vi "Dhoot Front Coordinate Sys.vi"(0 "Image Out":T8, 1 "First Reference ROI":T7={"Left"=660.0, "Top"=360.0, "Right"=900.0, "Bottom"=560.0, "Angle"=0.0}, 2 "Second Reference ROI":T7={"Left"=700.0, "Top"=200.0, "Right"=670.0, "Bottom"=0.0, "Angle"=0.0}, 3 "Options":T6={"Search Direction"=2, "Edge Options"={"Edge Polarity"=0, "Kernel Size"=7, "Width"=7, "Minimum Edge Strength"=40.0, "Interpolation Type"=enum."Zero Order", "Data Processing Method"=enum."Average"}, "Show Search Area"=FALSE, "Show Search Lines"=FALSE, "Show Edges Found"=FALSE, "Show Result"=TRUE, "Search Area Color"=65280, "Search Lines Color"=255, "Edge Locations Color"=16776960, "Result Color"=16711680, "Overlay Group Name"=""} {"Search Direction" items=["Left to Right", "Right to Left", "Top to Bottom", "Bottom to Top"]; "Edge Options"."Edge Polarity" items=["All Edges", "Rising Edges", "Falling Edges"]; "Edge Options"."Minimum Edge Strength" format="%.2f"; "Edge Options"."Width" step=2; "Edge Options"."Kernel Size" step=2}, 4 "Line Fit Options":T4={"Number of Lines"=1, "Type"=enum."First Edge Rake", "Min. Score"=10.0, "Max. Score"=1000.0, "Orientation"=0.0, "Angle Range"=45.0, "Angle Tolerance"=1.0, "Step Size"=7, "Min. SNR (db)"=0.0, "Min. Points (%)"=25.0, "Hough Iterations"=5} {"Min. Points (%)" min=0.0 max=100.0; "Min. SNR (db)" min=0.0; "Max. Score" min=0.0 max=1024.0; "Min. Score" min=0.0 max=1024.0 step=1.0}, 5 "error in (no error)":errorcluster, 6 "Edge Options":T1={"Edge Polarity"=0, "Kernel Size"=5, "Width"=5, "Minimum Edge Strength"=40.0, "Interpolation Type"=enum."Zero Order", "Data Processing Method"=enum."Average"} {"Edge Polarity" items=["All Edges", "Rising Edges", "Falling Edges"]; "Minimum Edge Strength" format="%.2f"; "Width" step=2; "Kernel Size" step=2}, 7 "ROI Enable True/False":bool, 8 "Step Size":u32=1, 9 "Process":T3(ring)=enum."Get First + Last Edge", 11 "Scan Direction":u16(ring) items=["Left To Right", "Right To Left", "Top To Bottom", "Bottom To Top"]) -> (13 "Angle (Pixel)":dbl, 14 "Image Out":T8, 15 "First Reference Centre":cluster{"Centre X":dbl, "Centre Y":dbl}, 16 "Second Reference Centre":cluster{"Centre X":dbl, "Centre Y":dbl}, 19 "error IO":errorcluster)   [LabVIEW 2019, in "Algorithm.lvclass"]
uses:
  FrameworkOverrides/Algorithm.lvclass
  <vilib>/vision/NI_Vision_Development_Module.lvlib
  <vilib>/vision/Image Controls.llb/IMAQ Image.ctl
  <vilib>/vision/Measure.llb/Edge Polarity.ctl
  <vilib>/vision/Measure.llb/Edge Options.ctl
  <vilib>/vision/Measure.llb/Straight Edge Process.ctl
  <vilib>/vision/Measure.llb/Straight Edge Options.ctl
panel:
  out "First ref Centre Y":dbl
  out "First ref Centre X":dbl
  out "Second ref Centre Y":dbl
  out "Second ref Centre X":dbl
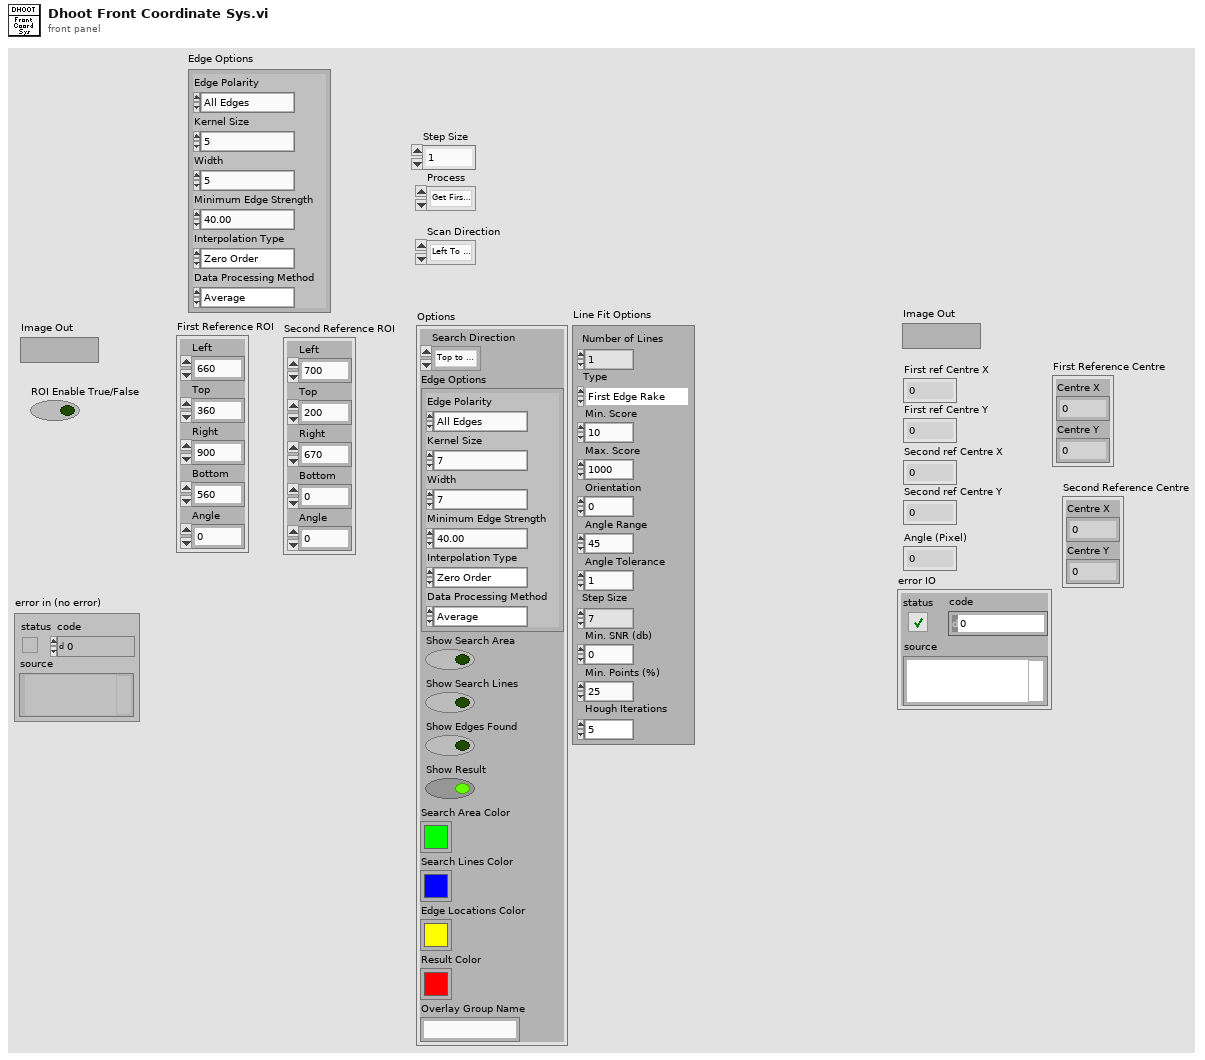
[diagram p1: front panel]
types:
  T1 = typedef "Edge Options.ctl" = cluster{"Edge Polarity":T2, "Kernel Size":u32, "Width":u32, "Minimum Edge Strength":sgl, "Interpolation Type":enum32{"Zero Order", "Bilinear", "Quadratic", "Cubic", "Bilinear Fixed"}, "Data Processing Method":enum32{"Average", "Median"}}
  T2 = typedef "Edge Polarity.ctl" = u32
  T3 = enum16{"Get First Edge", "Get First + Last Edge", "Get All Edges", "Get Best Edge"}
  T4 = typedef "Straight Edge Options.ctl" = cluster{"Number of Lines":i32, "Type":T5, "Min. Score":dbl, "Max. Score":dbl, "Orientation":dbl, "Angle Range":dbl, "Angle Tolerance":dbl, "Step Size":u32, "Min. SNR (db)":dbl, "Min. Points (%)":dbl, "Hough Iterations":i32}
  T5 = typedef "Straight Edge Process.ctl" = enum32{"First Edge Rake", "Best Edge Rake", "Hough Edge Rake", "First Edge Projection", "Best Edge Projection"}
  T6 = cluster{"Search Direction":u32, "Edge Options":T1, "Show Search Area":bool, "Show Search Lines":bool, "Show Edges Found":bool, "Show Result":bool, "Search Area Color":u32, "Search Lines Color":u32, "Edge Locations Color":u32, "Result Color":u32, "Overlay Group Name":string}
  T7 = cluster{"Left":dbl, "Top":dbl, "Right":dbl, "Bottom":dbl, "Angle":dbl}
  T8 = typedef "IMAQ Image.ctl" = refnum<image>
  T9 = typedef "ROI Descriptor" = cluster{"Global Rectangle":i32[], "Contours":cluster{"ID":enum32{"External", "Internal"}, "Type":u32, "Coordinates":i32[]}[]}
  T10 = cluster{"Point1 (Pixels)":cluster{"X":sgl, "Y":sgl}, "Point2 (Pixels)":cluster{"X":sgl, "Y":sgl}, "Point1 (Real-World)":cluster{"X":sgl, "Y":sgl}, "Point2 (Real-World)":cluster{"X":sgl, "Y":sgl}, "Angle (Pixel)":dbl, "Angle (Real-World)":dbl, "Score":dbl, "Straightness":dbl, "Average SNR (db)":dbl, "Calibration Valid":bool}[]
  T11 = cluster{"Point1 (Pixels)":cluster{"X":sgl, "Y":sgl}, "Point2 (Pixels)":cluster{"X":sgl, "Y":sgl}, "Point1 (Real-World)":cluster{"X":sgl, "Y":sgl}, "Point2 (Real-World)":cluster{"X":sgl, "Y":sgl}, "Angle (Pixel)":dbl, "Angle (Real-World)":dbl, "Score":dbl, "Straightness":dbl, "Average SNR (db)":dbl, "Calibration Valid":bool}
  T12 = typedef "Edge New.ctl" = cluster{"Location (Pixel)":cluster{"X":sgl, "Y":sgl}, "Location (Real-World)":cluster{"X":sgl, "Y":sgl}, "Distance (Pixel)":dbl, "Distance (Real-World)":dbl, "Strength":dbl, "Noise":dbl, "Rising?":bool}
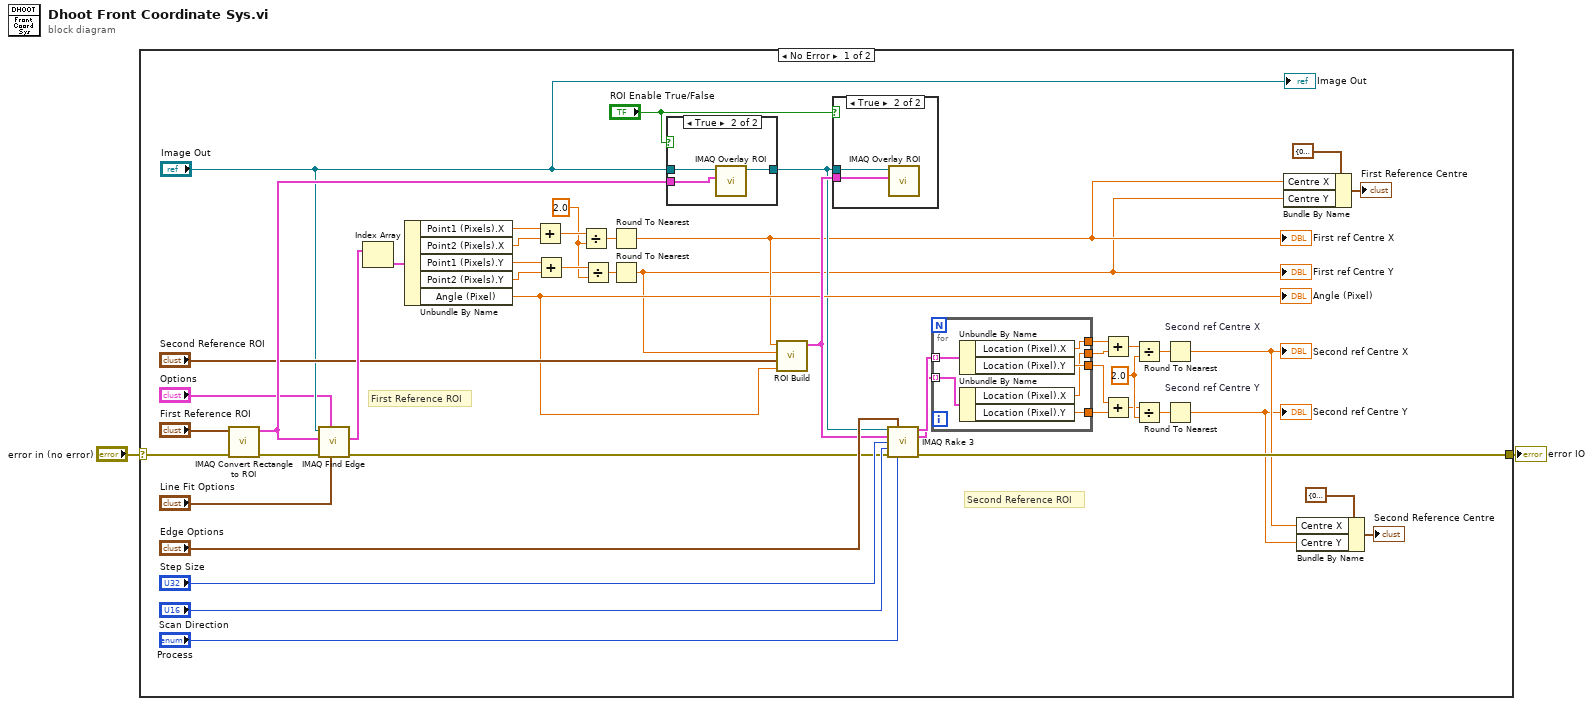
[diagram p0: block diagram]
diagram:
  n1 = case shown="No Error" "error in (no error)" {
    selector: "error in (no error)" -> [w14 w63]
    tunnel: [w13 w63] -> w1
    frame No Error {
      w25 = 2.0
      w39 = 2.0
      # "Second Reference ROI"
      # "First Reference ROI"
      n2 = call "IMAQ Convert Rectangle to ROI"("error in (no error)"=w14, "Rectangle"="First Reference ROI") -> ("error out"=w15:errorcluster, "ROI Descriptor"=w46:T9)  [unwired: 7 in]
      n3 = call "IMAQ Find Edge"("Line Fit Options"="Line Fit Options", "Options"="Options", "error in (no error)"=w15, "ROI Descriptor"=w46, "Image"="Image Out") -> ("error out"=w29:errorcluster, "Straight Edges"=w49:T10)  [unwired: 3 in, 2 out]
      n4 = Index Array(array=w49) -> (element=w48:T11)  [unwired: 1 in]
      n5 = Unbundle By Name(w48) -> ("Point1 (Pixels).X"=w45:sgl, "Point2 (Pixels).X"=w44:sgl, "Point1 (Pixels).Y"=w43:sgl, "Point2 (Pixels).Y"=w42:sgl, "Angle (Pixel)"=w22:dbl)
      "Angle (Pixel)" <- w22
      n6 = Add(x=w45, y=w44) -> (x+y=w41:sgl)
      n7 = Add(x=w43, y=w42) -> (x+y=w40:sgl)
      n8 = Divide(x=w41, y=w39) -> (x/y=w38:dbl)
      n9 = Divide(x=w40, y=w39) -> (x/y=w37:dbl)
      n10 = Round To Nearest(number=w38) -> (nearest integer value=w10:dbl)
      "First ref Centre X" <- w10
      n11 = Round To Nearest(number=w37) -> (nearest integer value=w9:dbl)
      "First ref Centre Y" <- w9
      n12 = case shown="True" "ROI Enable True/False" {
        tunnel: w46 -> [_ w56]
        tunnel: "Image Out" -> [w53 w55]
        tunnel: [w53 w54] -> w17
        frame False {
        }
        frame True {
          n13 = call "IMAQ Overlay ROI"("ROI Descriptor"=w56, "Image"=w55) -> ("Image Out"=w54:T8)  [unwired: 8 in, 1 out]
        }
      }
      n14 = call "ROI Build.vi"("Angle"=w22, "input cluster"="Second Reference ROI", "Centre Y"=w9, "Centre X"=w10) -> ("ROI Descriptor"=w30:T9)  [unwired: 7 in]
      n15 = case shown="True" "ROI Enable True/False" {
        tunnel: w30 -> [_ w52]
        tunnel: w17 -> [_ w51]
        frame False {
        }
        frame True {
          n16 = call "IMAQ Overlay ROI"("ROI Descriptor"=w52, "Image"=w51) -> ()  [unwired: 8 in, 2 out]
        }
      }
      n17 = call "IMAQ Rake 3"("Image"=w17, "Edge Options"="Edge Options", "ROI Descriptor"=w30, "Step Size"="Step Size", "Scan Direction"="Scan Direction", "error in (no error)"=w29, "Process"="Process") -> ("First Edges"=w31:T12[], "Last Edges"=w28:T12[], "error out"=w13:errorcluster)  [unwired: 5 in, 1 out]
      n18 = for {
        tunnel: w31 -> [w62] mode=indexing
        tunnel: w28 -> [w61] mode=indexing
        tunnel: [w60] -> w21
        tunnel: [w59] -> w19
        tunnel: [w58] -> w20
        tunnel: [w57] -> w18
        n19 = Unbundle By Name(w62) -> ("Location (Pixel).X"=w60:sgl, "Location (Pixel).Y"=w59:sgl)
        n20 = Unbundle By Name(w61) -> ("Location (Pixel).X"=w58:sgl, "Location (Pixel).Y"=w57:sgl)
      }
      n21 = Add(x=w21, y=w20) -> (x+y=w23:sgl)
      n22 = Add(x=w19, y=w18) -> (x+y=w24:sgl)
      n23 = Divide(x=w23, y=w25) -> (x/y=w26:dbl)
      n24 = Divide(x=w24, y=w25) -> (x/y=w27:dbl)
      n25 = Round To Nearest "Second ref Centre X"(number=w26) -> (nearest integer value=w4:dbl)
      "Second ref Centre X" <- w4
      n26 = Round To Nearest "Second ref Centre Y"(number=w27) -> (nearest integer value=w3:dbl)
      "Second ref Centre Y" <- w3
      n27 = Bundle By Name(cluster=cluster{"Centre X":dbl, "Centre Y":dbl} {"Centre X"=0.0, "Centre Y"=0.0} ("output cluster"), "Centre X"=w10, "Centre Y"=w9) -> (→"First Reference Centre":cluster{"Centre X":dbl, "Centre Y":dbl})
      n28 = Bundle By Name(cluster=cluster{"Centre X":dbl, "Centre Y":dbl} {"Centre X"=0.0, "Centre Y"=0.0} ("output cluster"), "Centre X"=w4, "Centre Y"=w3) -> (→"Second Reference Centre":cluster{"Centre X":dbl, "Centre Y":dbl})
      "Image Out" <- "Image Out"
    }
    frame Error {
    }
  }
  "error IO" <- w1
